vi "image.vi"(0 "Camera in":refnum<class "Camera.lvclass">, 5 "data_format":T3(ring)=enum."Mono16", 7 "image_index":u32, 9 "crop":cluster{"x0":u64, "y0":u64, "x1":u64, "y1":u64}={"x0"=1, "y0"=1, "x1"=18446744073709551615, "y1"=18446744073709551615}, 11 "error in (no error)":errorcluster, 12 "PCO_Recorder_CompressionParams":T5={"dGainK"=nan, "dDarkNoise_e"=nan, "dDSNU_e"=nan, "dPRNU_pct"=nan, "dLightSourceNoise_pct"=0.0}) -> (2 "timestamp":T4 {"lvTimestamp" format="%<%.6X\n%x>T"}, 3 "meta_data":T1, 4 "Camera out":refnum<class "Camera.lvclass">, 6 "image (U8)":u8[][](array[numeric]), 8 "image (U32)":u32[][](array[numeric]), 10 "image (U64)":T2(array[cluster]), 13 "raw_image_8bit (U8)":u8[][](array[numeric]), 14 "raw_image (U16)":u16[][](array[numeric]), 15 "error out":errorcluster)   [LabVIEW 2019, in "Camera.lvclass"]
doc: "Get an image from the recorder. The type of the image is 2D array of pixel values. This array is shaped depending on the resolution and ROI of the image. The data format determines which output is valid, but the raw_image(16) output is always valid."
uses:
  Camera.lvclass
  Camera.lvclass/Camera.ctl
  pco.recorder/Recorder.lvlib
  pco.convert/Convert.lvlib
panel:
  out "rawFormat":enum16{"Word", "Byte"}(ring)
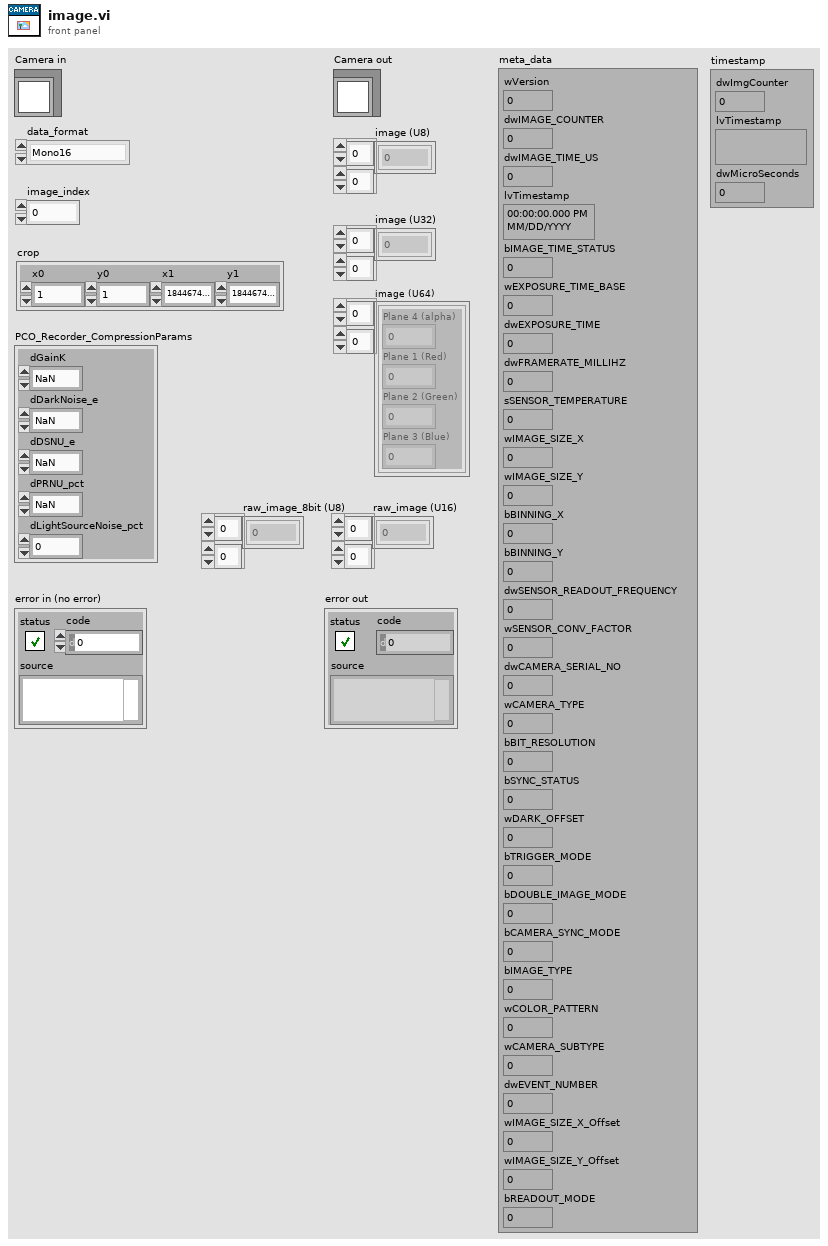
[diagram p1: front panel]
types:
  T1 = cluster{"wVersion":u16, "dwIMAGE_COUNTER":u32, "dwIMAGE_TIME_US":u32, "lvTimestamp":timestamp, "bIMAGE_TIME_STATUS":u8, "wEXPOSURE_TIME_BASE":u16, "dwEXPOSURE_TIME":u32, "dwFRAMERATE_MILLIHZ":u32, "sSENSOR_TEMPERATURE":i16, "wIMAGE_SIZE_X":u16, "wIMAGE_SIZE_Y":u16, "bBINNING_X":u8, "bBINNING_Y":u8, "dwSENSOR_READOUT_FREQUENCY":u32, "wSENSOR_CONV_FACTOR":u16, "dwCAMERA_SERIAL_NO":u32, "wCAMERA_TYPE":u16, "bBIT_RESOLUTION":u8, "bSYNC_STATUS":u8, "wDARK_OFFSET":u16, "bTRIGGER_MODE":u8, "bDOUBLE_IMAGE_MODE":u8, "bCAMERA_SYNC_MODE":u8, "bIMAGE_TYPE":u8, "wCOLOR_PATTERN":u16, "wCAMERA_SUBTYPE":u16, "dwEVENT_NUMBER":u32, "wIMAGE_SIZE_X_Offset":u16, "wIMAGE_SIZE_Y_Offset":u16, "bREADOUT_MODE":u8}
  T2 = cluster{"Plane 4 (alpha)":u16, "Plane 1 (Red)":u16, "Plane 2 (Green)":u16, "Plane 3 (Blue)":u16}[][]
  T3 = enum16{"Undefined", "Mono8", "Mono16", "BGRA8", "RGBA8", "BGRA16", "RGBA16", "CompressedMono8"}
  T4 = cluster{"dwImgCounter":u32, "lvTimestamp":timestamp, "dwMicroSeconds":u32}
  T5 = cluster{"dGainK":dbl, "dDarkNoise_e":dbl, "dDSNU_e":dbl, "dPRNU_pct":dbl, "dLightSourceNoise_pct":dbl}
  T6 = map{enum16{"Undefined", "Mono8", "Mono16", "BGRA8", "RGBA8", "BGRA16", "RGBA16", "CompressedMono8"}, cluster{"sharpen":bool, "adaptive_sharpen":bool, "flip_vertical":bool, "auto_minmax":bool, "add_conv_flags":u32, "min_limit":u16, "max_limit":u16, "gamma":dbl, "contrast":i32, "pco_debayer_algorithm":bool, "color_temperature":i32, "color_saturation":i32, "color_vibrance":i32, "color_tint":i32, "lut_file":path}}
  T7 = map{enum16{"Undefined", "Mono8", "Mono16", "BGRA8", "RGBA8", "BGRA16", "RGBA16", "CompressedMono8"}, bool}
  T8 = cluster{"sharpen":bool, "adaptive_sharpen":bool, "flip_vertical":bool, "auto_minmax":bool, "add_conv_flags":u32, "min_limit":u16, "max_limit":u16, "gamma":dbl, "contrast":i32, "pco_debayer_algorithm":bool, "color_temperature":i32, "color_saturation":i32, "color_vibrance":i32, "color_tint":i32, "lut_file":path}
  T9 = map{enum16{"Undefined", "Mono8", "Mono16", "BGRA8", "RGBA8", "BGRA16", "RGBA16", "CompressedMono8"}, u64}
  T10 = cluster{"Blue":u16, "Green":u16, "Red":u16, "Alpha":u16}[][]
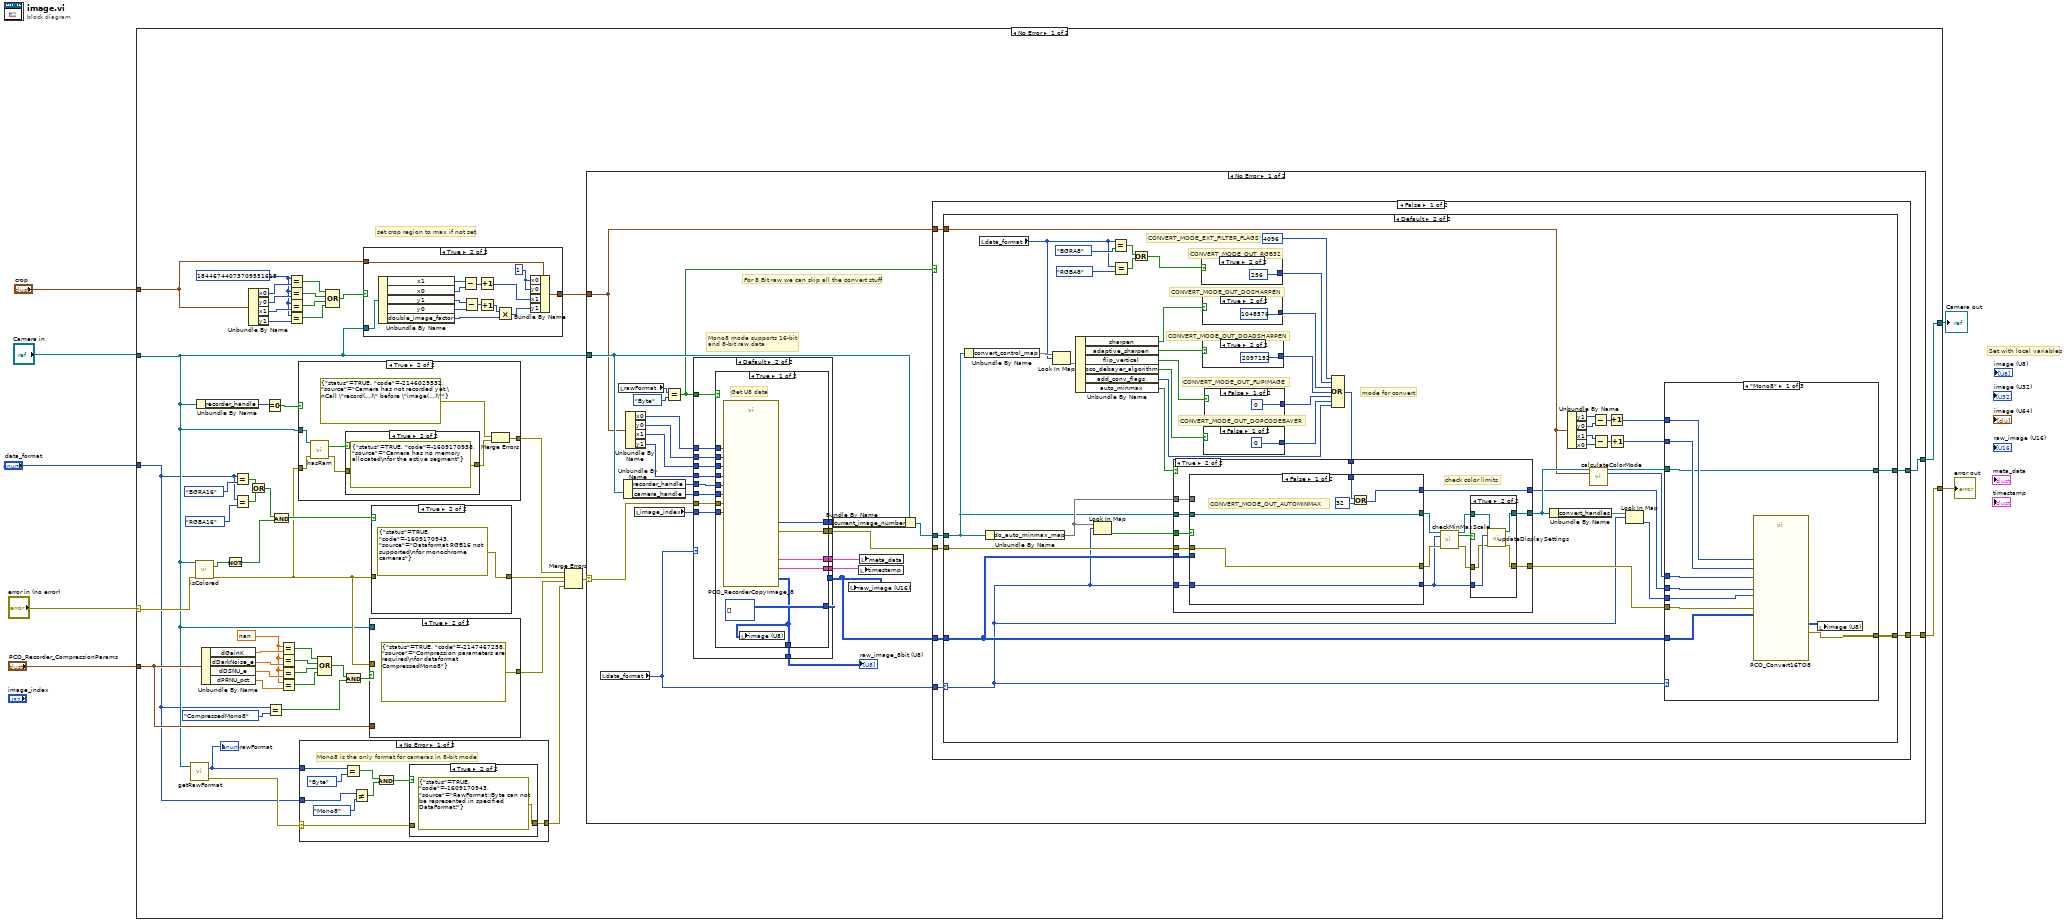
[diagram p0: block diagram]
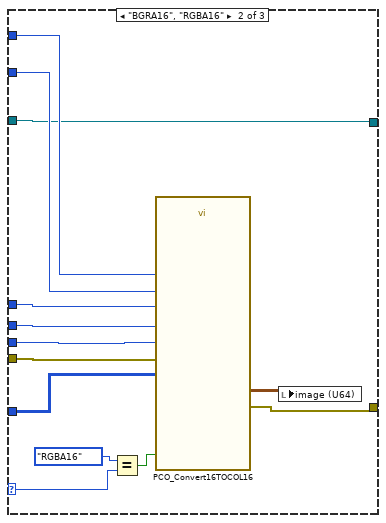
[diagram p6: hidden frame]
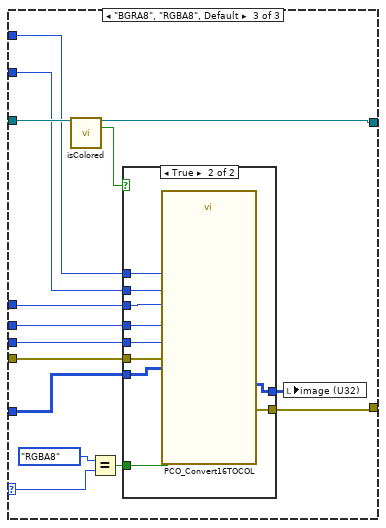
[diagram p7: hidden frame]
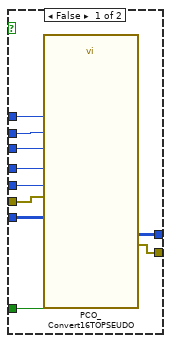
[diagram p8: hidden frame]
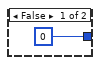
[diagram p9: hidden frame]
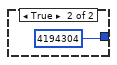
[diagram p10: hidden frame]
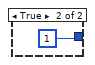
[diagram p11: hidden frame]
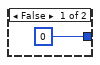
[diagram p12: hidden frame]
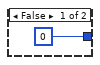
[diagram p13: hidden frame]
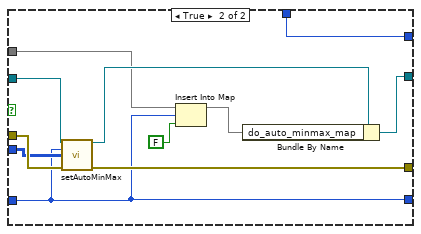
[diagram p16: hidden frame]
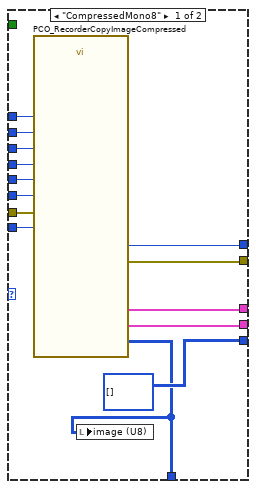
[diagram p18: hidden frame]
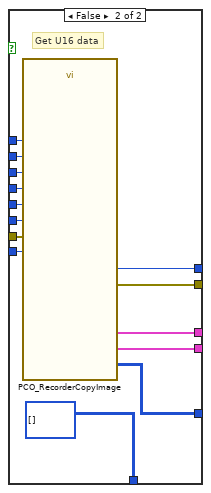
[diagram p19: hidden frame]
diagram:
  # "Set with local variables"
  n1 = case shown="No Error" "error in (no error)" {
    selector: "error in (no error)" -> [w56 w353]
    tunnel: [w22 w353] -> w6
    tunnel: [w23 w352] -> w4
    tunnel: "Camera in" -> [w12 w352]
    tunnel: "data_format" -> [w9 _]
    tunnel: "PCO_Recorder_CompressionParams" -> [w24 _]
    tunnel: "crop" -> [w20 _]
    frame No Error {
      w26 = u64 18446744073709551615 ("x0")
      w46 = nan ("dGainK")
      # "set crop region to max if not set"
      n2 = call-dynamic "getRawFormat.vi"("Camera in"=w12) -> ("rawFormat"=w10:enum16{"Word", "Byte"}, "error out"=w11:errorcluster)  [unwired: 12 in, 1 out]
      "rawFormat" <- w10
      n3 = call-dynamic "isColored.vi"("Camera in"=w12, "error in (no error)"=w56) -> ("colored"=w55:bool, "error out"=w38:errorcluster)  [unwired: 11 in, 1 out]
      n4 = Unbundle By Name(w12) -> ("recorder_handle"=w52:u64)
      n5 = Unbundle By Name(w24) -> ("dGainK"=w50:dbl, "dDarkNoise_e"=w49:dbl, "dDSNU_e"=w48:dbl, "dPRNU_pct"=w47:dbl)
      n6 = Not(x=w55) -> (.not. x?=w54:bool)
      n7 = Equal?(x=w9, y=T3."BGRA16" ("data_format")) -> (x = y?=w16:bool)
      n8 = Equal?(x=w9, y=T3."RGBA16" ("data_format")) -> (x = y?=w15:bool)
      n9 = Unbundle By Name(w20) -> ("x0"=w30:u64, "y0"=w29:u64, "x1"=w28:u64, "y1"=w27:u64)
      n10 = Or(x=w16, y=w15) -> (x .or. y?=w14:bool)
      n11 = Equal To 0?(x=w52) -> (x = 0?=w51:bool)
      n12 = Equal?(x=w9, y=T3."CompressedMono8" ("data_format")) -> (x = y?=w40:bool)
      n13 = And(x=w14, y=w54) -> (x .and. y?=w53:bool)
      n14 = Equal?(x=w46, y=w50) -> (x = y?=w45:bool)
      n15 = Equal?(x=w46, y=w49) -> (x = y?=w44:bool)
      n16 = Equal?(x=w46, y=w48) -> (x = y?=w43:bool)
      n17 = Equal?(x=w46, y=w47) -> (x = y?=w42:bool)
      n18 = Equal?(x=w26, y=w30) -> (x = y?=w31:bool)
      n19 = Equal?(x=w26, y=w29) -> (x = y?=w32:bool)
      n20 = Equal?(x=w26, y=w28) -> (x = y?=w33:bool)
      n21 = Equal?(x=w26, y=w27) -> (x = y?=w34:bool)
      n22 = case shown="True" w51 {
        tunnel: w38 -> [w333 w339]
        tunnel: [w333 w334] -> w37
        tunnel: w12 -> [_ w340]
        frame False {
        }
        frame True {
          n23 = call-dynamic "hasRam.vi"("Camera in"=w340, "error in (no error)"=w339) -> ("hasRam"=w338:bool, "error out"=w337:errorcluster)  [unwired: 11 in, 1 out]
          n24 = case shown="True" w338 {
            tunnel: w337 -> [w341 _]
            tunnel: [w341 errorcluster {"status"=TRUE, "code"=-1609170938, "source"="Camera has no memory allocated\nfor the active segment"} ("error constant")] -> w335
            frame False {
            }
            frame True {
            }
          }
          n25 = Merge Errors(errorcluster {"status"=TRUE, "code"=-2146029532, "source"="Camera has not recorded yet.\nCall \"record(...)\" before \"image(...)\""} ("error constant"), w335) -> (w334:errorcluster)
        }
      }
      n26 = case shown="No Error" w11 {
        selector: w11 -> [w58 w68]
        tunnel: w10 -> [w65 _]
        tunnel: w9 -> [w63 _]
        tunnel: [w57 w68] -> w8
        frame No Error {
          # "Mono8 is the only format for cameras in 8-bit mode"
          n27 = Equal?(x=w65, y=enum16{"Word", "Byte"}."Byte" ("rawFormat")) -> (x = y?=w61:bool)
          n28 = Not Equal?(x=w63, y=T3."Mono8" ("data_format")) -> (x != y?=w60:bool)
          n29 = And(x=w61, y=w60) -> (x .and. y?=w59:bool)
          n30 = case shown="True" w59 {
            tunnel: w58 -> [w66 _]
            tunnel: [w66 errorcluster {"status"=TRUE, "code"=-1609170943, "source"="RawFormat::Byte can not be represented in specified DataFormat!"} ("error constant")] -> w57
            frame False {
            }
            frame True {
            }
          }
        }
        frame Error {
        }
      }
      n31 = Compound Arithmetic op=OR(w45, w44, w43, w42) -> (w41:bool)
      n32 = Compound Arithmetic op=OR(w31, w32, w33, w34) -> (w21:bool)
      n33 = And(x=w41, y=w40) -> (x .and. y?=w39:bool)
      n34 = case shown="True" w21 {
        tunnel: w12 -> [_ w83]
        tunnel: w20 -> [w69 w82]
        tunnel: [w69 w81] -> w19
        frame False {
        }
        frame True {
          w80 = u16 1 ("x0")
          n35 = Unbundle By Name(w83) -> ("x1"=w79:u64, "x0"=w78:u64, "y1"=w76:u64, "y0"=w75:u64, "double_image_factor"=w71:u16)
          n36 = Subtract(x=w79, y=w78) -> (x-y=w77:u64)
          n37 = Subtract(x=w76, y=w75) -> (x-y=w73:u64)
          n38 = Increment(x=w77) -> (x+1=w74:u64)
          n39 = Increment(x=w73) -> (x+1=w72:u64)
          n40 = Multiply(x=w72, y=w71) -> (x*y=w70:u64)
          n41 = Bundle By Name(cluster=w82, "x0"=w80, "y0"=w80, "x1"=w74, "y1"=w70) -> (w81:cluster{"x0":u64, "y0":u64, "x1":u64, "y1":u64})
        }
      }
      n42 = case shown="True" w39 {
        tunnel: [w345 errorcluster {"status"=TRUE, "code"=-2147467258, "source"="Compression parameters are required\nfor dataformat CompressedMono8"} ("error constant")] -> w35
        tunnel: w38 -> [w350 _]
        tunnel: w24 -> [w346 _]
        tunnel: w12 -> [w349 _]
        frame False {
          n43 = Unbundle By Name(w349) -> ("recorder_handle"=w348:u64, "camera_handle"=w347:u64)
          n44 = call "PCO_RecorderSetCompressionParams.vi"("phRec"=w348, "phCam"=w347, "strCompressionParams"=w346, "error in (no error)"=w350) -> ("error out"=w345:errorcluster)  [unwired: 9 in, 2 out]
        }
        frame True {
        }
      }
      n45 = case shown="True" w53 {
        tunnel: w38 -> [w343 _]
        tunnel: [w343 errorcluster {"status"=TRUE, "code"=-1609170943, "source"="Dataformat RGB16 not supported\nfor monochrome cameras"} ("error constant")] -> w36
        frame False {
        }
        frame True {
        }
      }
      n46 = Merge Errors(w37, w36, w35, w8) -> (w25:errorcluster)
      n47 = case shown="No Error" w25 {
        selector: w25 -> [w97 w332]
        tunnel: w19 -> [w92 _]
        tunnel: w12 -> [w96 w331]
        tunnel: [w91 w331] -> w23
        tunnel: [w90 w332] -> w22
        frame No Error {
          # "For 8 Bit raw we can skip all the convert stuff"
          # "Mono8 mode supports 16-bit and 8-bit raw data"
          n48 = local read "data_format"() -> (w89:T3)
          n49 = local read "rawFormat"() -> (w88:enum16{"Word", "Byte"})
          n50 = Unbundle By Name(w96) -> ("recorder_handle"=w102:u64, "camera_handle"=w103:u64)
          n51 = Unbundle By Name(w92) -> ("x0"=w98:u64, "y0"=w99:u64, "x1"=w100:u64, "y1"=w101:u64)
          n52 = local read "image_index"() -> (w104:u32)
          n53 = Equal?(x=w88, y=enum16{"Word", "Byte"}."Byte" ("rawFormat")) -> (x = y?=w85:bool)
          n54 = case shown="Default" w89 {
            tunnel: [w279 w302] -> w106
            tunnel: [w277 w301] -> w84
            tunnel: [w276 w300] -> w105
            tunnel: w104 -> [w280 w299]
            tunnel: w103 -> [w282 w298]
            tunnel: w102 -> [w283 w297]
            tunnel: w101 -> [w284 w296]
            tunnel: w100 -> [w285 w295]
            tunnel: w99 -> [w286 w294]
            tunnel: w98 -> [w287 w293]
            tunnel: w97 -> [w281 w292]
            tunnel: [u16[][] [] ("wImgBuf") w289] -> w95
            tunnel: [w278 w291] -> w94
            tunnel: [w274 w290] -> w86
            tunnel: w85 -> [_ w288]
            frame "CompressedMono8" {
              n55 = call "PCO_RecorderCopyImageCompressed.vi"("phRec"=w283, "phCam"=w282, "dwImgIdx"=w280, "wRoiX0"=w287, "wRoiY0"=w286, "wRoiX1"=w285, "wRoiY1"=w284, "error in (no error)"=w281) -> ("strTimestamp"=w276:T4, "strMetadata"=w277:T1, "bImgBuf"=w274:u8[][], "dwImgNumber"=w279:u32, "error out"=w278:errorcluster)  [unwired: 13 in, 2 out]
              n56 = local write "image (U8)"(w274) -> ()
            }
            frame Default {
              n57 = case shown="True" w288 {
                tunnel: [w316 w330] -> w302
                tunnel: [w315 w329] -> w301
                tunnel: [w314 w328] -> w300
                tunnel: w299 -> [w313 w327]
                tunnel: w298 -> [w312 w326]
                tunnel: w297 -> [w311 w325]
                tunnel: w296 -> [w310 w324]
                tunnel: w295 -> [w309 w323]
                tunnel: w294 -> [w308 w322]
                tunnel: w293 -> [w307 w321]
                tunnel: w292 -> [w306 w320]
                tunnel: [w305 w319] -> w291
                tunnel: [w303 u8[][] []] -> w290
                tunnel: [u16[][] [] w318] -> w289
                frame True {
                  # "Get U8 data"
                  n58 = call "PCO_RecorderCopyImage_8.vi"("phRec"=w311, "phCam"=w312, "dwImgIdx"=w313, "wRoiX0"=w307, "wRoiY0"=w308, "wRoiX1"=w309, "wRoiY1"=w310, "error in (no error)"=w306) -> ("strTimestamp"=w314:T4, "strMetadata"=w315:T1, "bImgBuf"=w303:u8[][], "dwImgNumber"=w316:u32, "error out"=w305:errorcluster)  [unwired: 13 in, 2 out]
                  n59 = local write "image (U8)"(w303) -> ()
                }
                frame False {
                  # "Get U16 data"
                  n60 = call "PCO_RecorderCopyImage.vi"("phRec"=w325, "phCam"=w326, "dwImgIdx"=w327, "wRoiX0"=w321, "wRoiY0"=w322, "wRoiX1"=w323, "wRoiY1"=w324, "error in (no error)"=w320) -> ("strTimestamp"=w328:T4, "strMetadata"=w329:T1, "wImgBuf"=w318:u16[][], "dwImgNumber"=w330:u32, "error out"=w319:errorcluster)  [unwired: 13 in, 2 out]
                }
              }
            }
          }
          "raw_image_8bit (U8)" <- w86
          n61 = Bundle By Name(cluster=w96, "current_image_number"=w106) -> (w93:refnum<class "Camera.lvclass">)
          n62 = local write "raw_image (U16)"(w95) -> ()
          n63 = local write "timestamp"(w105) -> ()
          n64 = local write "meta_data"(w84) -> ()
          n65 = case shown="False" w85 {
            tunnel: w95 -> [w113 _]
            tunnel: w94 -> [w112 w273]
            tunnel: w93 -> [w111 w272]
            tunnel: w92 -> [w110 _]
            tunnel: [w109 w272] -> w91
            tunnel: [w108 w273] -> w90
            tunnel: w89 -> [w107 _]
            frame False {
              n66 = case shown="Default" w107 {
                selector: w107 -> [_ w118]
                tunnel: w112 -> [w114 w160]
                tunnel: w113 -> [_ w147]
                tunnel: w111 -> [w115 w137]
                tunnel: w110 -> [_ w157]
                tunnel: [w115 w142] -> w109
                tunnel: [w114 w141] -> w108
                frame "Mono16", "CompressedMono8" {
                }
                frame Default {
                  # "CONVERT_MODE_OUT_RGB32"
                  # "CONVERT_MODE_OUT_FLIPIMAGE"
                  # "CONVERT_MODE_OUT_DOPCODEBAYER"
                  # "CONVERT_MODE_OUT_DOADSHARPEN"
                  # "CONVERT_MODE_OUT_DOSHARPEN"
                  # "CONVERT_MODE_EXT_FILTER_FLAGS"
                  # "mode for convert"
                  n67 = Unbundle By Name(w137) -> ("convert_control_map"=w136:T6)
                  n68 = local read "data_format"() -> (w123:T3)
                  n69 = Unbundle By Name(w137) -> ("do_auto_minmax_map"=w139:T7)
                  n70 = Look In Map(map=w136, key=w123) -> (value=w135:T8)  [unwired: 1 in, 1 out]
                  n71 = Unbundle By Name(w135) -> ("sharpen"=w134:bool, "adaptive_sharpen"=w133:bool, "flip_vertical"=w125:bool, "pco_debayer_algorithm"=w132:bool, "add_conv_flags"=w116:u32, "auto_minmax"=w117:bool)
                  n72 = Look In Map(map=w139, key=w118) -> (value=w140:bool)  [unwired: 1 in, 1 out]
                  n73 = Equal?(x=w123, y=T3."BGRA8" ("data_format")) -> (x = y?=w121:bool)
                  n74 = Equal?(x=w123, y=T3."RGBA8" ("data_format")) -> (x = y?=w120:bool)
                  n75 = Or(x=w121, y=w120) -> (x .or. y?=w119:bool)
                  n76 = case shown="True" w119 {
                    tunnel: [u32 0 ("image_index") u32 256 ("image_index")] -> w126
                    frame False {
                    }
                    frame True {
                    }
                  }
                  n77 = case shown="True" w134 {
                    tunnel: [u32 0 ("image_index") u32 1048576 ("image_index")] -> w131
                    frame False {
                    }
                    frame True {
                    }
                  }
                  n78 = case shown="True" w133 {
                    tunnel: [u32 0 ("image_index") u32 2097152 ("image_index")] -> w130
                    frame False {
                    }
                    frame True {
                    }
                  }
                  n79 = case shown="False" w132 {
                    tunnel: [u32 0 ("image_index") u32 4194304 ("image_index")] -> w128
                    frame False {
                    }
                    frame True {
                    }
                  }
                  n80 = case shown="False" w125 {
                    tunnel: [u32 0 ("image_index") u32 1 ("image_index")] -> w129
                    frame False {
                    }
                    frame True {
                    }
                  }
                  n81 = Compound Arithmetic op=OR(u32 4096 ("image_index"), w126, w131, w130, w129, w128, w116) -> (w138:u32)
                  n82 = case shown="True" w117 {
                    tunnel: w160 -> [w230 w247]
                    tunnel: [w231 w234] -> w158
                    tunnel: [w229 w246] -> w149
                    tunnel: w147 -> [_ w245]
                    tunnel: [w230 w233] -> w144
                    tunnel: w140 -> [_ w244]
                    tunnel: w139 -> [_ w243]
                    tunnel: w138 -> [w229 w242]
                    tunnel: w137 -> [w231 w241]
                    tunnel: w118 -> [_ w240]
                    frame False {
                    }
                    frame True {
                      # "check color limits"
                      n83 = case shown="False" w244 {
                        tunnel: w241 -> [w256 w271]
                        tunnel: w242 -> [w258 w263]
                        tunnel: [w257 w263] -> w246
                        tunnel: w245 -> [_ w262]
                        tunnel: w240 -> [w255 w261]
                        tunnel: [w256 w270] -> w239
                        tunnel: w247 -> [w260 w269]
                        tunnel: [w260 w268] -> w238
                        tunnel: w243 -> [_ w264]
                        tunnel: [w255 w261] -> w232
                        frame False {
                          # "CONVERT_MODE_OUT_AUTOMINMAX"
                          n84 = Or(x=w258, y=u32 32 ("image_index")) -> (x .or. y?=w257:u32)
                        }
                        frame True {
                          n85 = call-dynamic "setAutoMinMax.vi"("Camera in"=w271, "data_format"=w261, "image"=w262, "error in (no error)"=w269) -> ("Camera out"=w266:refnum<class "Camera.lvclass">, "error out"=w268:errorcluster)  [unwired: 10 in]
                          n86 = Insert Into Map(map in=w264, key=w261, value=FALSE) -> (map out=w265:T7)  [unwired: 2 out]
                          n87 = Bundle By Name(cluster=w266, "do_auto_minmax_map"=w265) -> (w270:refnum<class "Camera.lvclass">)
                        }
                      }
                      n88 = call-dynamic "checkMinMaxScale.vi"("Camera in"=w239, "data_format"=w232, "error in (no error)"=w238) -> ("Camera out"=w236:refnum<class "Camera.lvclass">, "needsUpdate"=w237:bool, "error out"=w235:errorcluster)  [unwired: 10 in]
                      n89 = case shown="True" w237 {
                        tunnel: w236 -> [w249 w254]
                        tunnel: w235 -> [w248 w250]
                        tunnel: [w249 w252] -> w234
                        tunnel: [w248 w253] -> w233
                        tunnel: w232 -> [_ w251]
                        frame False {
                        }
                        frame True {
                          n90 = call-dynamic "updateDisplaySettings.vi"("Camera in"=w254, "data_format"=w251, "error in (no error)"=w250) -> ("Camera out"=w252:refnum<class "Camera.lvclass">, "error out"=w253:errorcluster)  [unwired: 11 in]
                        }
                      }
                    }
                  }
                  n91 = Unbundle By Name(w158) -> ("convert_handles"=w159:T9)
                  n92 = Unbundle By Name(w157) -> ("y1"=w155:u64, "y0"=w156:u64, "x1"=w154:u64, "x0"=w153:u64)
                  n93 = call-dynamic "calculateColorMode.vi"("Camera in"=w158, "crop"=w157) -> ("Camera out"=w143:refnum<class "Camera.lvclass">, "colorMode"=w148:i32)  [unwired: 11 in, 1 out]
                  n94 = Subtract(x=w155, y=w156) -> (x-y=w152:u64)
                  n95 = Subtract(x=w154, y=w153) -> (x-y=w151:u64)
                  n96 = Increment(x=w152) -> (x+1=w146:u64)
                  n97 = Increment(x=w151) -> (x+1=w145:u64)
                  n98 = Look In Map(map=w159, key=w118) -> (value=w150:u64)  [unwired: 1 in, 1 out]
                  n99 = case shown="\"Mono8\"" w118 {
                    selector: w118 -> [_ w173 w185]
                    tunnel: w150 -> [w165 w178 w191]
                    tunnel: w149 -> [w166 w179 w188]
                    tunnel: w148 -> [w167 w180 w187]
                    tunnel: w147 -> [w163 w181 w197]
                    tunnel: w146 -> [w169 w183 w190]
                    tunnel: w145 -> [w168 w182 w189]
                    tunnel: w144 -> [w164 w177 w192]
                    tunnel: w143 -> [w161 w175 w196]
                    tunnel: [w161 w175 w194] -> w142
                    tunnel: [w162 w176 w195] -> w141
                    frame "Mono8" {
                      n100 = call "PCO_Convert16TO8.vi"("ph"=w165, "height"=w169, "mode"=w166, "icolmode"=w167, "width"=w168, "error in (no error)"=w164, "b16"=w163) -> ("b8"=w170:u8[][], "error out"=w162:errorcluster)  [unwired: 5 in, 2 out]
                      n101 = local write "image (U8)"(w170) -> ()
                    }
                    frame "BGRA16", "RGBA16" {
                      n102 = Equal?(x=T3."RGBA16" ("data_format"), y=w173) -> (x = y?=w172:bool)
                      n103 = call "PCO_Convert16TOCOL16.vi"("ph"=w178, "height"=w183, "swap_colors"=w172, "mode"=w179, "icolmode"=w180, "width"=w182, "error in (no error)"=w177, "raw_image(U16)"=w181) -> ("image (U64)"=w171:T10, "error out"=w176:errorcluster)  [unwired: 4 in, 2 out]
                      n104 = local write "image (U64)"(w171) -> ()
                    }
                    frame "BGRA8", "RGBA8", Default {
                      n105 = call-dynamic "isColored.vi"("Camera in"=w196) -> ("Camera out"=w194:refnum<class "Camera.lvclass">, "colored"=w198:bool)  [unwired: 12 in, 1 out]
                      n106 = Equal?(x=T3."RGBA8" ("data_format"), y=w185) -> (x = y?=w184:bool)
                      n107 = case shown="True" w198 {
                        tunnel: w197 -> [w206 w217]
                        tunnel: [w208 w218] -> w195
                        tunnel: [w207 w210] -> w193
                        tunnel: w192 -> [w205 w216]
                        tunnel: w191 -> [w204 w215]
                        tunnel: w190 -> [w200 w214]
                        tunnel: w189 -> [w201 w213]
                        tunnel: w188 -> [w203 w212]
                        tunnel: w187 -> [w202 w209]
                        tunnel: w184 -> [w199 w211]
                        frame False {
                          n108 = call "PCO_Convert16TOPSEUDO.vi"("ph"=w204, "height"=w200, "swap_colors"=w199, "mode"=w203, "icolmode"=w202, "width"=w201, "error in (no error)"=w205, "b16"=w206) -> ("b32"=w207:u32[][], "error out"=w208:errorcluster)  [unwired: 4 in, 2 out]
                        }
                        frame True {
                          n109 = call "PCO_Convert16TOCOL.vi"("ph"=w215, "height"=w214, "swap_colors"=w211, "mode"=w212, "icolmode"=w209, "width"=w213, "error in (no error)"=w216, "b16"=w217) -> ("b32"=w210:u32[][], "error out"=w218:errorcluster)  [unwired: 4 in, 2 out]
                        }
                      }
                      n110 = local write "image (U32)"(w193) -> ()
                    }
                  }
                }
              }
            }
            frame True {
            }
          }
        }
        frame Error {
        }
      }
    }
    frame Error {
    }
  }
  "error out" <- w6
  "Camera out" <- w4
